vi "SignalChange.vi"(11 "Signal":bool) -> (2 "T_to_F":bool, 3 "F_to_T":bool)   [LabVIEW 2017]
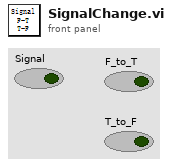
[diagram p1: front panel]
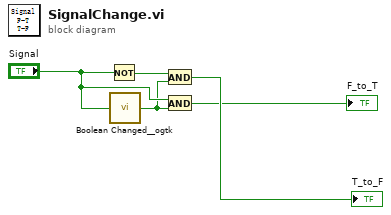
[diagram p0: block diagram]
diagram:
  n1 = Not(x="Signal") -> (.not. x?=w2:bool)
  n2 = call "Boolean Changed__ogtk.vi"("Boolean"="Signal") -> ("Changed"=w3:bool)
  n3 = And(x=w2, y=w3) -> (x .and. y?=→"T_to_F":bool)
  n4 = And(x="Signal", y=w3) -> (x .and. y?=→"F_to_T":bool)
